vi "Rcv Cmd.vi"(8 "error in":errorcluster, 11 "PAS in":refnum<class "PAS.lvclass">) -> (0 "error out":errorcluster, 3 "PAS out":refnum<class "PAS.lvclass">)   [LabVIEW 2014, in "PAS.lvclass"]
doc: "The override of the <b>Instrument:Rcv Cmd</b> method accounts for checking for speaker switching when the object is set to autocycle. How the change in switch state is executed is left to the <b>Change Speaker State</b> command object which is sent when the state is to be changed."
uses:
  PAS.lvclass
  PAS.lvclass/PAS.ctl
  PAS/Commands/Change Speaker State/Change Speaker State.lvclass
  Instrument/Instrument.lvclass/Instrument.ctl
  Instrument/Read CMD.vi
  Switch/Switch.lvclass
  Command/Command.lvclass
  Instrument/Instrument.lvclass
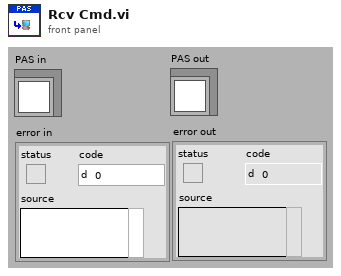
[diagram p1: front panel]
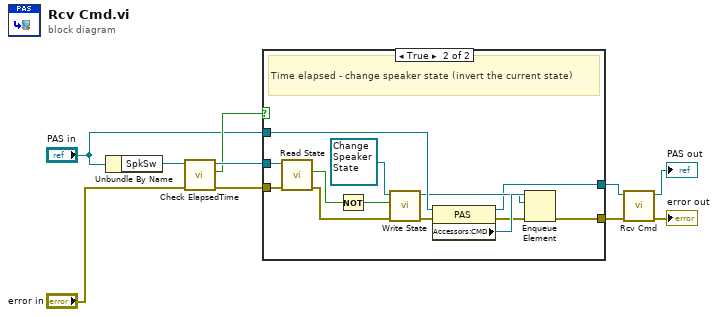
[diagram p0: block diagram]
diagram:
  n1 = Unbundle By Name("PAS in") -> ("SpkSw"=w8:refnum<class "Switch.lvclass">)
  n2 = call-dynamic "Check ElapsedTime.vi"("error in"="error in", "Switch in"=w8) -> ("error out"=w6:errorcluster, "Cycle Switch?"=w5:bool, "Switch out"=w7:refnum<class "Switch.lvclass">)  [unwired: 6 in, 1 out]
  n3 = case shown="True" w5 {
    tunnel: w7 -> [_ w25]
    tunnel: w6 -> [w11 w24]
    tunnel: "PAS in" -> [w12 w20]
    tunnel: [w12 w16] -> w3
    tunnel: [w11 w13] -> w2
    frame False {
    }
    frame True {
      # "Time elapsed - change speaker state (invert the current state)"
      n4 = call-dynamic "Read State.vi"("error in (no error)"=w24, "Switch in"=w25) -> ("error out"=w17:errorcluster, "State"=w21:bool)  [unwired: 7 in, 1 out]
      n5 = Not(x=w21) -> (.not. x?=w22:bool)
      n6 = call "Write State.vi"("error in (no error)"=w17, "State"=w22, "Change Speaker State in"=refnum<class "Change Speaker State.lvclass"> refnum ("Change Speaker State.lvclass")) -> ("error out"=w15:errorcluster, "Change Speaker State out"=w18:refnum<class "Change Speaker State.lvclass">)  [unwired: 7 in]
      n7 = property class="PAS"(reference=w20, error in=w15) -> (reference out=w16:refnum<class "PAS.lvclass">, error out=w14:errorcluster, "Accessors:CMD"=w19:refnum<queue>)
      n8 = Enqueue Element(queue=w19, element=w18, error in (no error)=w14) -> (error out=w13:errorcluster)  [unwired: 1 in, 2 out]
    }
  }
  n9 = call-parent "Rcv Cmd.vi"("error in"=w2, "Instrument in"=w3) -> ("error out"=→"error out":errorcluster, "Instrument out"=→"PAS out":refnum<class "PAS.lvclass">)  [unwired: 8 in]
